vi "prepareEvent.vi"(6 "cmdStatus":string(combo)="ack", 8 "error in (no error)":errorcluster, 10 "command":string, 11 "TcpServer in":refnum<class "TcpServer.lvclass">) -> (0 "error out":errorcluster, 2 "JSON string":string, 3 "TcpServer out":refnum<class "TcpServer.lvclass">)   [LabVIEW 2018]
doc: "Prepare the command received to make the Ack."
uses:
  TcpServer.lvclass
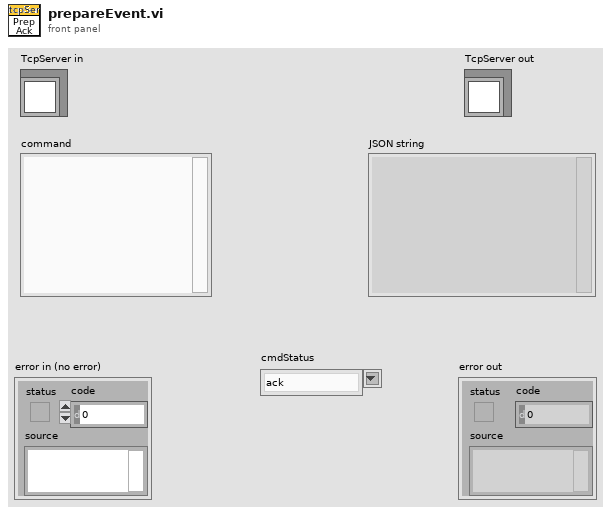
[diagram p1: front panel]
types:
  T1 = cluster{"cmdName":string, "cmdId":i32, "cmdStatus":string}
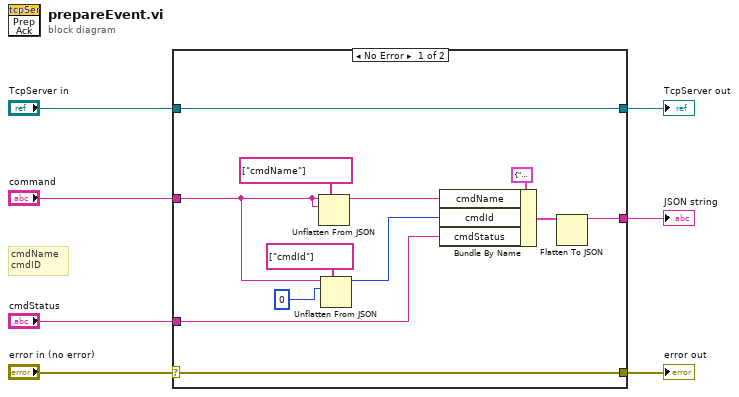
[diagram p0: block diagram]
diagram:
  # "cmdName\ncmdID"
  n1 = case shown="No Error" "error in (no error)" {
    selector: "error in (no error)" -> [w18 w21]
    tunnel: [w18 w21] -> w6
    tunnel: [w19 w20] -> w4
    tunnel: "TcpServer in" -> [w19 w20]
    tunnel: "command" -> [w15 _]
    tunnel: "cmdStatus" -> [w10 _]
    tunnel: [w8 _] -> w1
    frame No Error {
      n2 = Unflatten From JSON(path=string[] ["cmdName"], JSON string=w15, type and defaults=w15) -> (value=w12:string)  [unwired: 4 in, 1 out]
      n3 = Unflatten From JSON(path=string[] ["cmdId"], JSON string=w15, type and defaults=0) -> (value=w11:i32)  [unwired: 4 in, 1 out]
      n4 = Bundle By Name(cluster=T1 {"cmdName"="", "cmdId"=0, "cmdStatus"=""}, "cmdName"=w12, "cmdId"=w11, "cmdStatus"=w10) -> (w9:T1)
      n5 = Flatten To JSON(anything=w9) -> (JSON string=w8:string)  [unwired: 2 in, 1 out]
    }
    frame Error {
    }
  }
  "error out" <- w6
  "TcpServer out" <- w4
  "JSON string" <- w1
